vi "Release Enqueue Semaphore.vi"(0 "Semaphore Reference":T1) -> ()   [LabVIEW 2013]
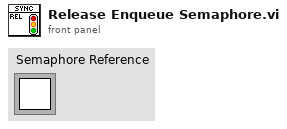
[diagram p1: front panel]
types:
  T1 = typedef "Semaphore RefNum" = refnum<k1>
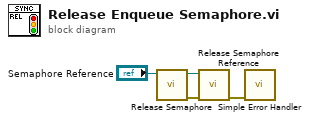
[diagram p0: block diagram]
diagram:
  n1 = call <vilib>:"Release Semaphore.vi"("semaphore"="Semaphore Reference") -> ("error out"=w4:errorcluster, "semaphore out"=w3:T1)  [unwired: 5 in]
  n2 = call <vilib>:"Release Semaphore Reference.vi"("error in (no error)"=w4, "semaphore"=w3) -> ("error out"=w2:errorcluster)  [unwired: 8 in, 1 out]
  n3 = call <vilib>:"Simple Error Handler.vi"("error in (no error)"=w2) -> ()  [unwired: 4 in, 5 out]
